vi "CTRL_Send Cmd.vi"(0 "Port":refnum<visa-resource-name>, 5 "RS-485 addr.":u8, 7 "Cmd":T1="D", 11 "Error In":errorcluster) -> (4 "Port out":refnum<visa-resource-name>, 15 "Error Out":errorcluster)   [LabVIEW 2020]
uses:
  ctls/CTRL_Cmd.ctl
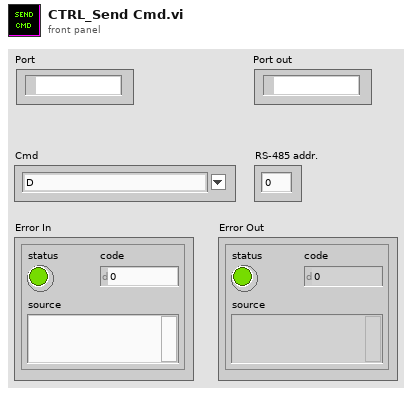
[diagram p1: front panel]
types:
  T1 = typedef "CTRL_Cmd.ctl" = string
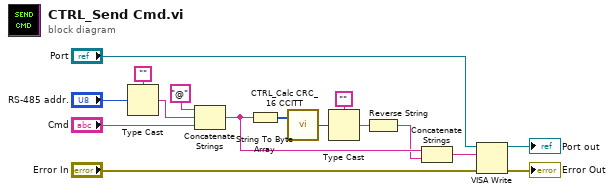
[diagram p0: block diagram]
diagram:
  n1 = Type Cast(type="", x="RS-485 addr.") -> (*(type *) &x=w2:string)
  n2 = Concatenate Strings("@", w2, "Cmd") -> (w6:string)
  n3 = String To Byte Array(string=w6) -> (unsigned byte array=w10:u8[])
  n4 = call "CTRL_Calc CRC_16 CCITT.vi"("Data bytes"=w10) -> ("CRC_16-CCITT"=w9:u16)  [unwired: 1 in]
  n5 = Type Cast(type="", x=w9) -> (*(type *) &x=w7:string)
  n6 = Reverse String(1:w7) -> (0:w1:string)
  n7 = Concatenate Strings(w6, w1) -> (w5:string)
  n8 = VISA Write(VISA resource name="Port", write buffer=w5, error in (no error)="Error In") -> (VISA resource name out=→"Port out":refnum<visa-resource-name>, error out=→"Error Out":errorcluster)  [unwired: 1 out]
